vi "Targets by Name.vi"(11 "Project Name":string) -> (2 "Targets":refnum<vi>[](array[refnum]), 3 "Project":refnum<vi>)   [LabVIEW 2020, in "Conditum-Tools.lvlib" / "Entity Editor.lvclass"]
uses:
  Entity Editor.lvclass
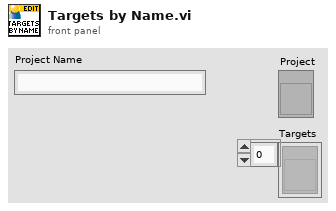
[diagram p1: front panel]
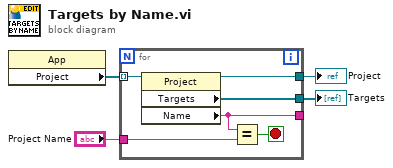
[diagram p0: block diagram]
diagram:
  n1 = property class="App"() -> ("Project"=w4:refnum<vi>[])  [unwired: 2 in, 2 out]
  n2 = for {
    tunnel: w4 -> [w10] mode=indexing
    tunnel: "Project Name" -> [w8]
    tunnel: [w9] -> w2
    tunnel: [w7] -> _
    tunnel: [w5] -> w1
    stop <- w6 stop-if-true
    n3 = property class="Project"(reference=w10) -> (reference out=w9:refnum<vi>, "Targets"=w5:refnum<vi>[], "Name"=w7:string)  [unwired: 1 in, 1 out]
    n4 = Equal?(x=w7, y=w8) -> (x = y?=w6:bool)
  }
  "Project" <- w2
  "Targets" <- w1
